vi "Raft_wars_Ver7.vi"() -> ()   [LabVIEW 2026]
panel:
  out "Computer Board":dbl[][](array[numeric])
  out "Player  Board":dbl[][](array[numeric])
  in  "Player Ship Inputs":T1(array[cluster]) {"Y-Coordinate" min=0 max=7; "X-Coordinate" min=0 max=7}
  in  "Emergency Stop":bool
  out "Game Status":string
  out "Ships Placed":dbl
  out "Losses":dbl
  out "Computer Hits":dbl
  out "Wins":dbl
  out "Player Hits":dbl
  in  "Attack":bool
  in  "Play Again":bool
  in  "Place Ship":bool
  in  "Attack Y":dbl
  in  "Attack X":dbl
  in  "Ship Y":dbl
  in  "Ship X":dbl
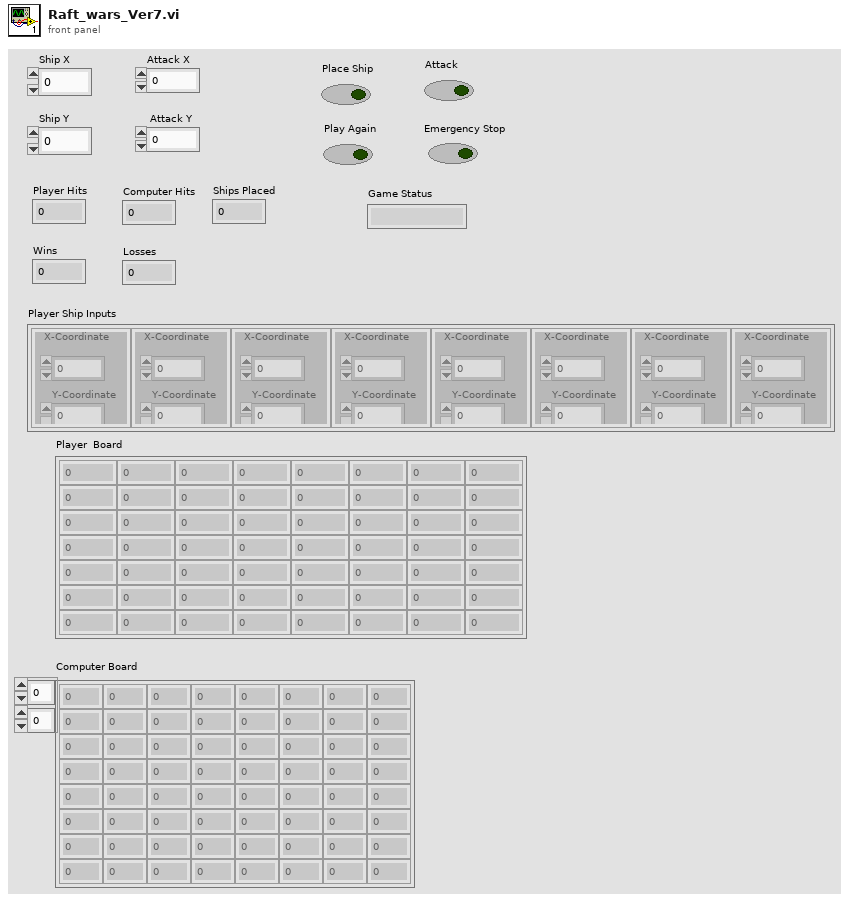
[diagram p1: front panel]
types:
  T1 = cluster{"X-Coordinate":i32, "Y-Coordinate":i32}[]
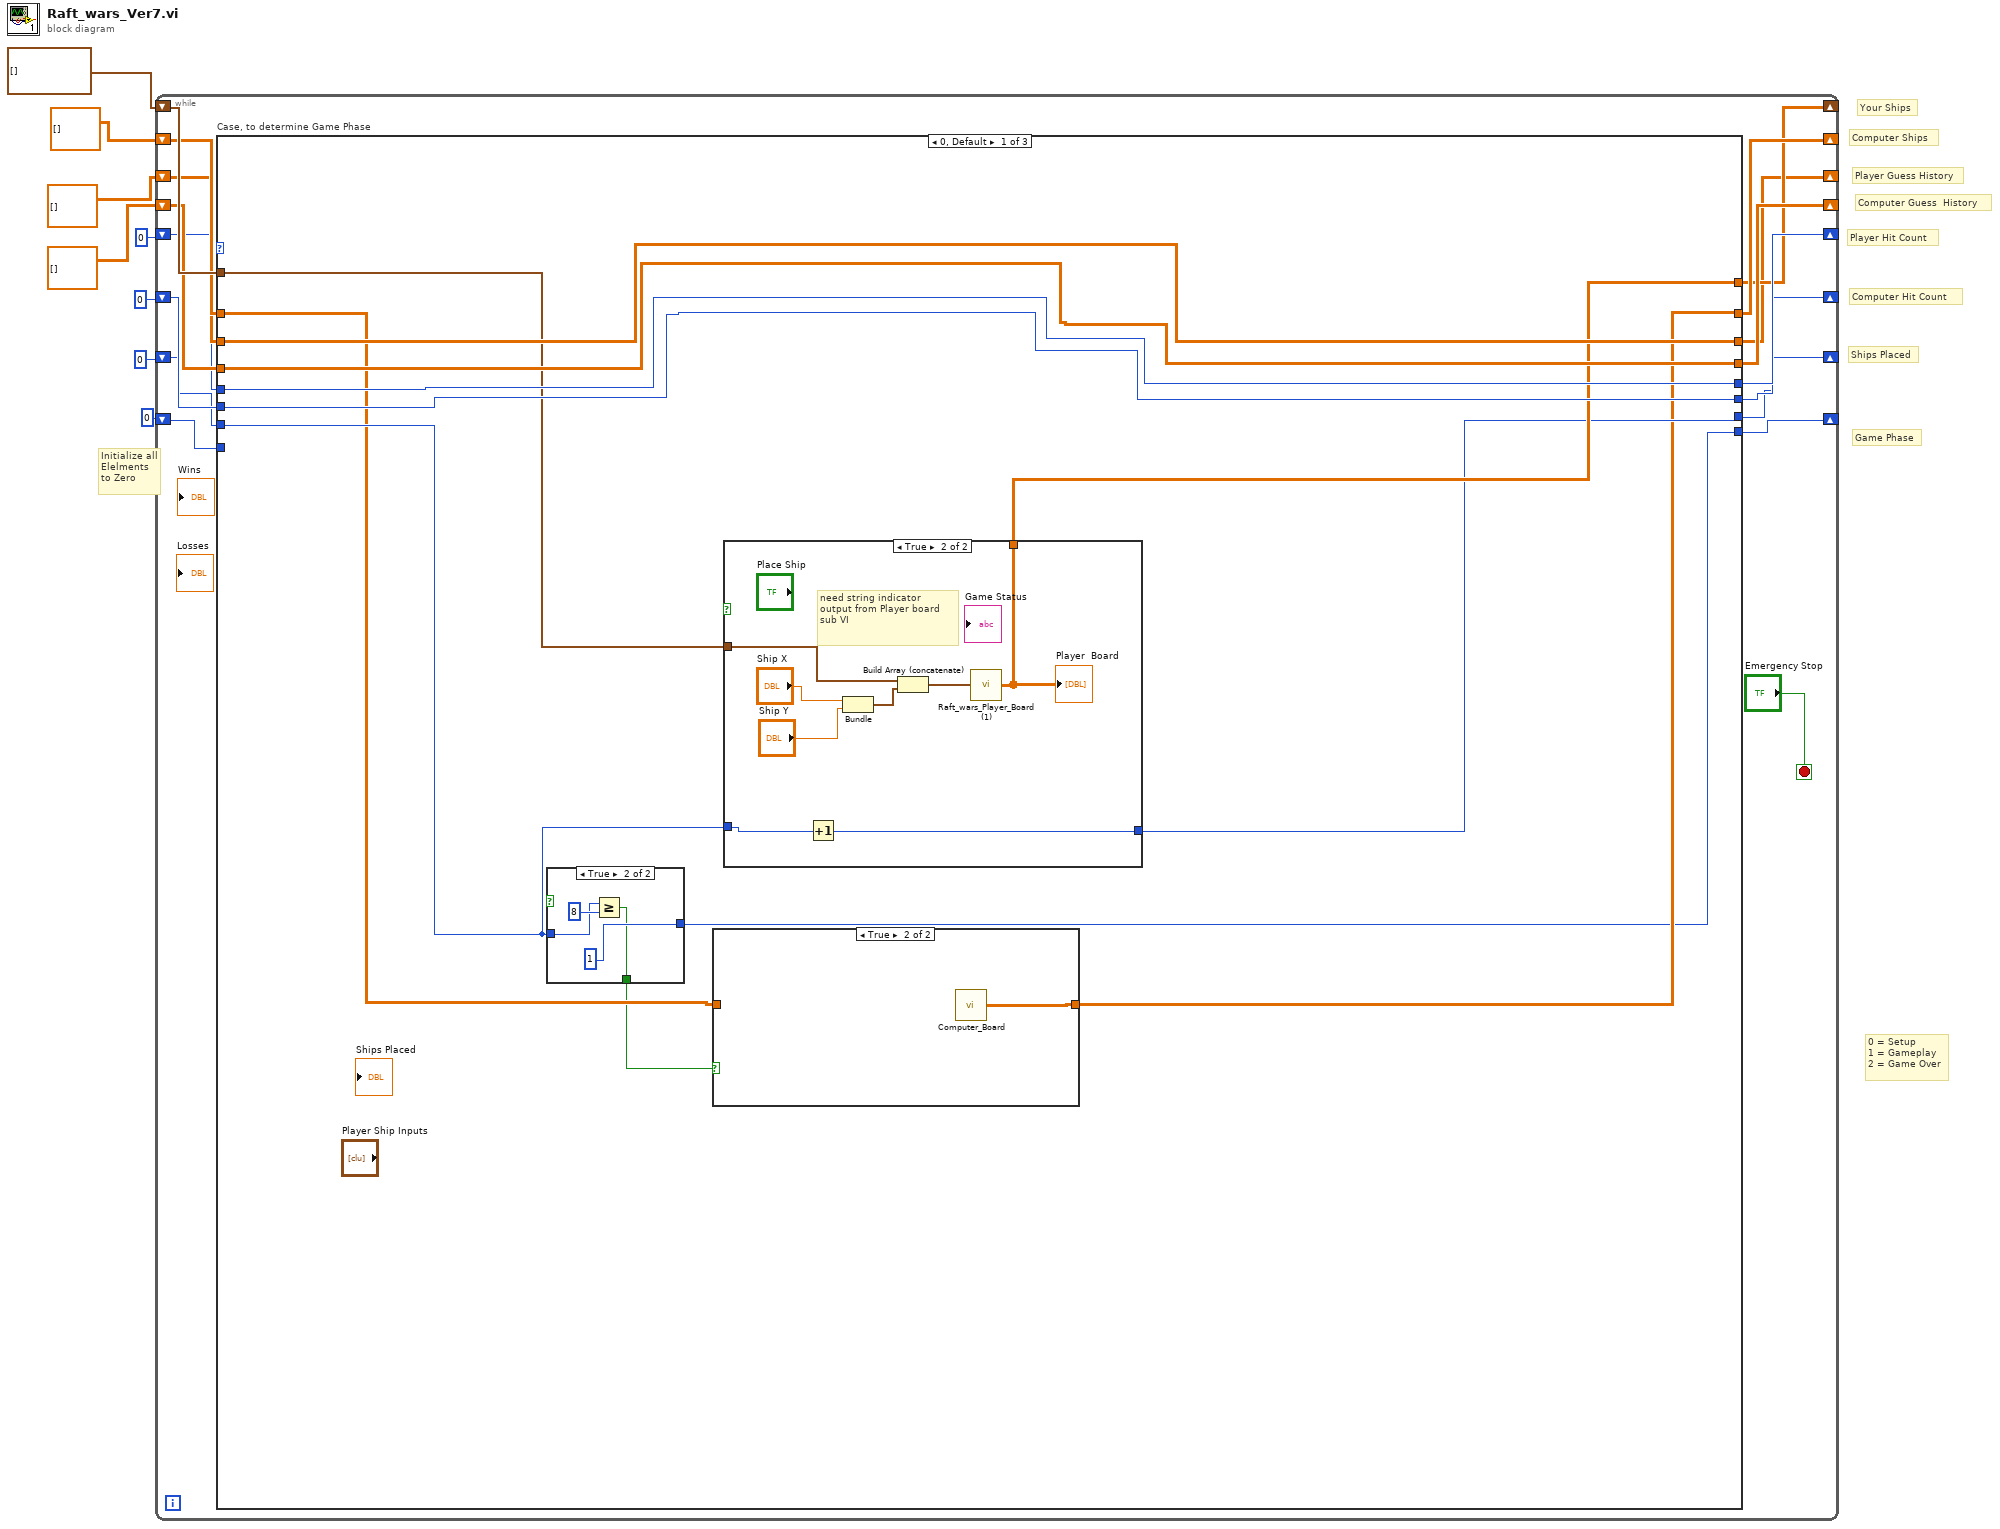
[diagram p0: block diagram]
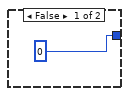
[diagram p3: hidden frame]
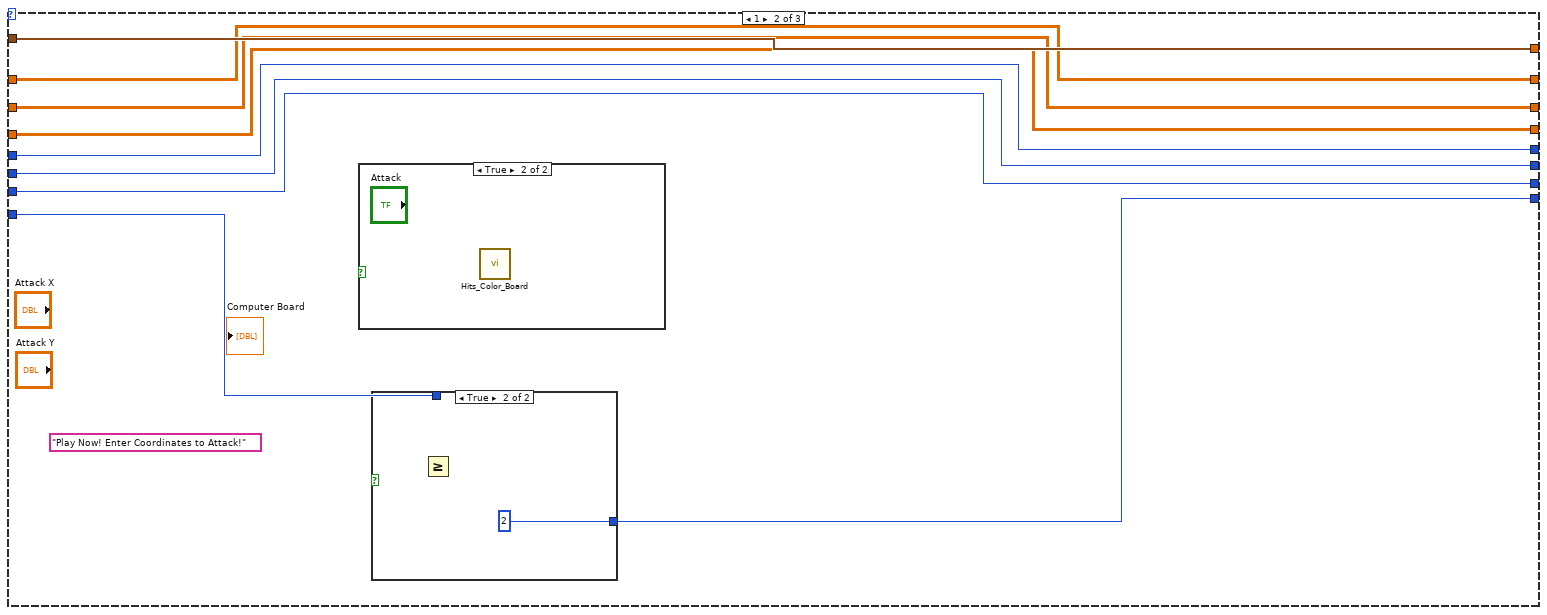
[diagram p5: hidden frame]
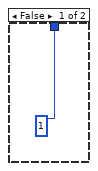
[diagram p6: hidden frame]
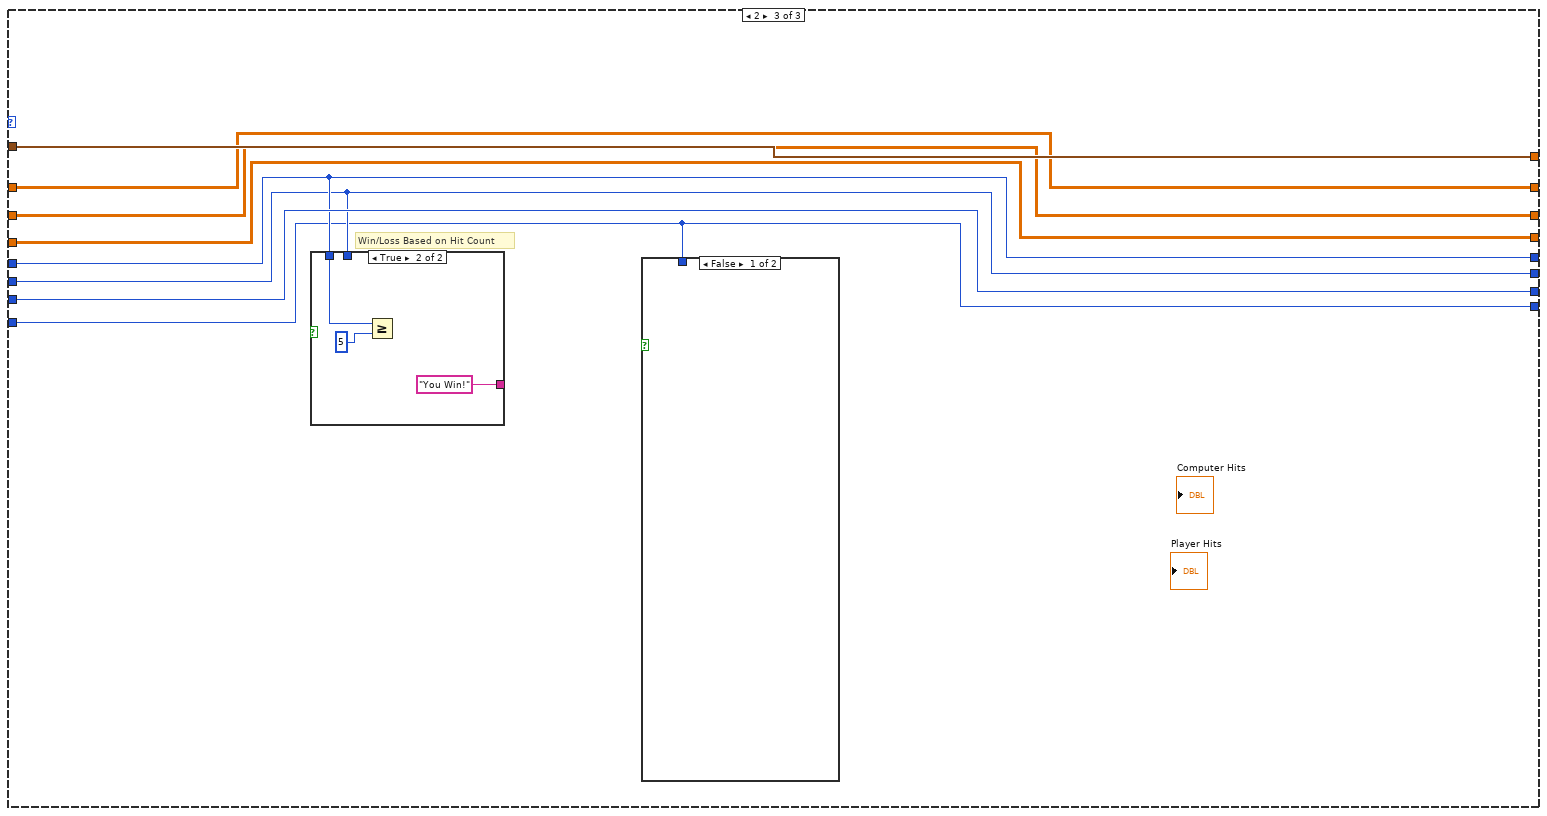
[diagram p8: hidden frame]
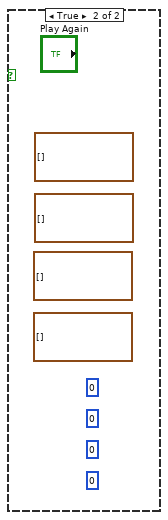
[diagram p9: hidden frame]
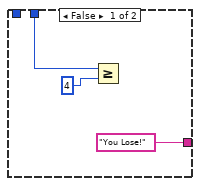
[diagram p10: hidden frame]
diagram:
  # "0 = Setup\n1 = Gameplay\n2 = Game Over"
  # "Initialize all\nElelments\nto Zero"
  # "Ships Placed"
  # "Your Ships"
  # "Computer Ships"
  # "Player Guess History"
  # "Computer Guess  History"
  # "Player Hit Count"
  # "Computer Hit Count"
  # "Game Phase"
  n1 = while {
    shift-right: [w10] -> _
    shift-left: cluster{i32, i32}[] [] -> [w24]
    shift-right: [w11] -> _
    shift-left: dbl[][] [] ("Array") -> [w23]
    shift-right: [w9] -> _
    shift-left: dbl[][] [] ("Array") -> [w22]
    shift-right: [w20] -> _
    shift-left: dbl[][] [] ("Array") -> [w21]
    shift-right: [w15] -> _
    shift-left: 0 -> [w19]
    shift-right: [w14] -> _
    shift-left: 0 -> [w18]
    shift-right: [w13] -> _
    shift-left: 0 -> [w17]
    shift-right: [w12] -> _
    shift-left: 0 -> [w16]
    stop <- "Emergency Stop" stop-if-true
    n2 = case "Case, to determine Game Phase" shown="0, Default" {
      selector: _ -> [_ _ _]
      tunnel: w24 -> [w33 w63 w73]
      tunnel: [w31 w63 w73] -> w10
      tunnel: w23 -> [w27 w58 w72]
      tunnel: [w29 w58 w72] -> w11
      tunnel: w22 -> [w37 w57 w71]
      tunnel: [w37 w57 w71] -> w9
      tunnel: w21 -> [w36 w62 w70]
      tunnel: [w36 w62 w70] -> w20
      tunnel: w19 -> [w35 w60 w68]
      tunnel: w18 -> [w34 w59 w67]
      tunnel: w17 -> [w32 w61 w69]
      tunnel: w16 -> [_ w55 w66]
      tunnel: [w35 w60 w68] -> w15
      tunnel: [w34 w59 w67] -> w14
      tunnel: [w30 w61 w69] -> w13
      tunnel: [w28 w56 w66] -> w12
      frame 0, Default {
        n3 = case shown="True" {
          selector: _ -> [_ _]
          tunnel: w32 -> [_ w43]
          tunnel: [0 1] -> w28
          tunnel: [_ w41] -> w26
          frame False {
          }
          frame True {
            n4 = Greater Or Equal?(x=w43, y=8) -> (x >= y?=w41:bool)
          }
        }
        n5 = case shown="True" w26 {
          tunnel: w27 -> [w38 _]
          tunnel: [w38 w39] -> w29
          frame False {
          }
          frame True {
            n6 = call "Computer_Board.vi"() -> ("Array"=w39:dbl[][])
          }
        }
        n7 = case shown="True" {
          selector: _ -> [_ _]
          tunnel: w33 -> [w46 w50]
          tunnel: w32 -> [w45 w48]
          tunnel: [w46 w49] -> w31
          tunnel: [w45 w47] -> w30
          frame False {
          }
          frame True {
            # "need string indicator\noutput from Player board \nsub VI"
            n8 = Increment(x=w48) -> (x+1=w47:i32)
            n9 = Bundle("Ship X"="Ship X", "Ship Y"="Ship Y") -> (w52:cluster{"Ship X":dbl, "Ship Y":dbl})  [unwired: 1 in]
            n10 = Build Array (concatenate)(w50, w52) -> (w51:cluster{"Ship X":dbl, "Ship Y":dbl}[])
            n11 = call "Raft_wars_Player_Board (1).vi"("Player Ship Inputs"=w51) -> ("Array"=w49:dbl[][])
            "Player  Board" <- w49
          }
        }
      }
      frame 1 {
        (unwired) "Play Now! Enter Coordinates to Attack!"
        n12 = case shown="True" {
          selector: _ -> [_ _]
          frame False {
          }
          frame True {
            n13 = call "Hits_Color_Board.vi"() -> ()  [unwired: 12 in]
          }
        }
        n14 = case shown="True" {
          selector: _ -> [_ _]
          tunnel: [_ 2] -> w56
          tunnel: [1 _] -> w55
          frame False {
          }
          frame True {
            n15 = Greater Or Equal?() -> ()  [unwired: 2 in, 1 out]
          }
        }
      }
      frame 2 {
        # "Win/Loss Based on Hit Count"
        n16 = case shown="True" {
          selector: _ -> [_ _]
          tunnel: w68 -> [_ w79]
          tunnel: ["You Lose!" "You Win!"] -> _
          tunnel: w67 -> [w74 _]
          frame False {
            n17 = Greater Or Equal?(x=w74, y=4) -> ()  [unwired: 1 out]
          }
          frame True {
            n18 = Greater Or Equal?(x=w79, y=5) -> ()  [unwired: 1 out]
          }
        }
        n19 = case shown="False" {
          selector: _ -> [_ _]
          tunnel: w66 -> [_ _]
          frame False {
          }
          frame True {
            (unwired) 0
            (unwired) 0
            (unwired) 0
            (unwired) cluster{dbl, dbl}[] []
            (unwired) cluster{dbl, dbl}[] []
            (unwired) cluster{dbl, dbl}[] []
            (unwired) cluster{dbl, dbl}[] []
            (unwired) 0
          }
        }
      }
    }
  }
